vi "Create DAQmx Task.vi"(8 "error in (no error)":errorcluster, 11 "DAQmxAI in":refnum<class "DAQmxAI.lvclass">) -> (0 "error out":errorcluster, 3 "DAQmxAI out":refnum<class "DAQmxAI.lvclass">)   [LabVIEW 2020, in "VolatusDAQ.lvlib" / "DAQmxAI.lvclass"]
uses:
  DAQmxAI.lvclass
  DAQmxAI.lvclass/DAQmxAI.ctl
  <vilib>/DAQmx/configure/timing.llb/DAQmx Timing (Sample Clock).vi
  VolatusDAQConfig/DAQmxChannel/DAQmxChannel.lvclass
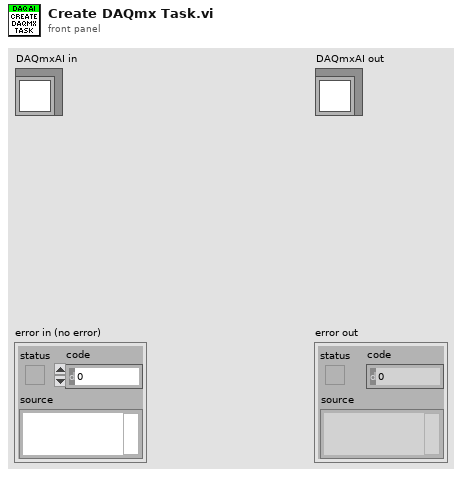
[diagram p1: front panel]
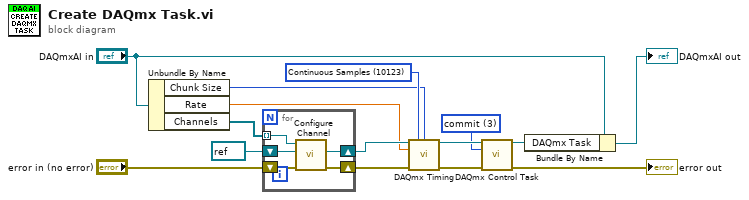
[diagram p0: block diagram]
diagram:
  w4 = 3 items=["verify"=2, "reserve"=4, "commit"=3, "unreserve"=5, "abort"=6] ("action")
  w9 = 10123 items=["Finite Samples"=10178, "Continuous Samples"=10123, "Hardware Timed Single Point"=12522] ("sample mode")
  n1 = Unbundle By Name("DAQmxAI in") -> ("Chunk Size"=w8:i32, "Rate"=w7:dbl, "Channels"=w13:refnum<class "DAQmxChannel.lvclass">[])
  n2 = for {
    shift-right: [w18] -> w11
    shift-left: refnum<k21> refnum ("DAQmx Task Name") -> [w19]
    tunnel: w13 -> [w20] mode=indexing
    shift-right: [w16] -> w10
    shift-left: "error in (no error)" -> [w17]
    n3 = call-dynamic "Configure Channel.vi"("error in (no error)"=w17, "DAQmx Task In"=w19, "DAQmxChannel in"=w20) -> ("error out"=w16:errorcluster, "DAQmx Task"=w18:refnum<k21>)  [unwired: 7 in]
  }
  n4 = call-poly <vilib>:"DAQmx Timing.vi"("task/channels in"=w11, "sample mode"=w9, "samples per channel"=w8, "rate"=w7, "error in"=w10) -> ("task out"=w5:refnum<k21>, "error out"=w6:errorcluster)  [unwired: 9 in]
  n5 = call <vilib>:"DAQmx Control Task.vi"("task/channels in"=w5, "action"=w4, "error in"=w6) -> ("task out"=w1:refnum<k21>, "error out"=→"error out":errorcluster)  [unwired: 11 in]
  n6 = Bundle By Name(cluster="DAQmxAI in", "DAQmx Task"=w1) -> (→"DAQmxAI out":refnum<class "DAQmxAI.lvclass">)
